vi "DSF.Engine.Execution.Builder.Get Plugin Buffer Pools.vi"(8 "error in (no error)":errorcluster, 11 "Builder in":refnum<class "DSF.Engine.Execution.Builder.lvclass">) -> (0 "error out":errorcluster, 2 "Plugin Buffer Pools":refnum<class "DSF.Engine.Memory.BufferPool.lvclass">[](array[class]), 3 "Builder out":refnum<class "DSF.Engine.Execution.Builder.lvclass">)   [LabVIEW 2016, in "DSF.Engine.lvlib" / "DSF.Engine.Execution.Builder.lvclass"]
uses:
  Builder/DSF.Engine.Execution.Builder.lvclass
  BufferPool/DSF.Engine.Memory.BufferPool.lvclass
  Builder/DSF.Engine.Execution.Builder.lvclass/DSF.Engine.Execution.Builder.ctl
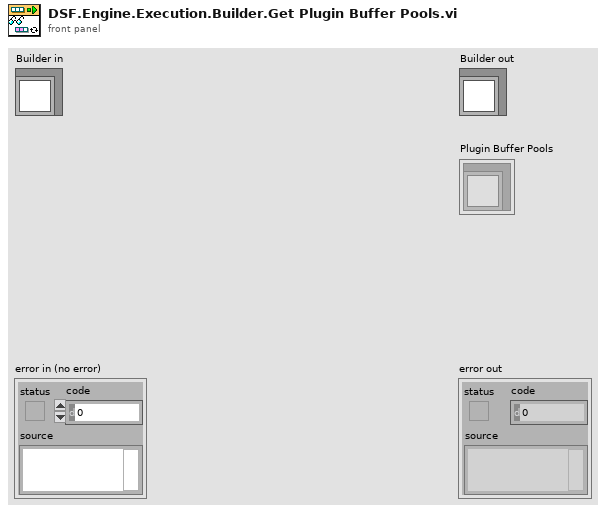
[diagram p1: front panel]
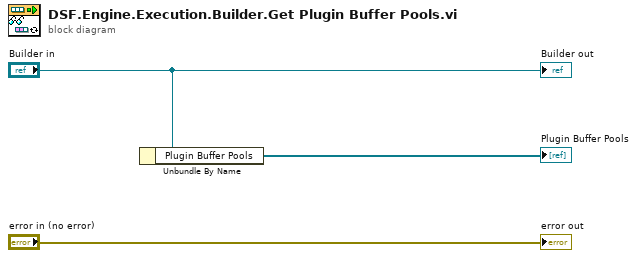
[diagram p0: block diagram]
diagram:
  n1 = Unbundle By Name("Builder in") -> ("Plugin Buffer Pools"=→"Plugin Buffer Pools":refnum<class "DSF.Engine.Memory.BufferPool.lvclass">[])
  "error out" <- "error in (no error)"
  "Builder out" <- "Builder in"
